vi "Read Frequency Response Analysis Data.vi"(8 "error in (no error)":errorcluster, 10 "Maximum Time (10000)":u32=10000, 11 "VISA resource name":refnum<visa-resource-name>) -> (0 "error out":errorcluster, 2 "Frequency Analysis Data":dbl[][](array[numeric]), 3 "VISA resource name out":refnum<visa-resource-name>)   [LabVIEW 2017, in "Agilent 2000 3000 X-Series.lvlib"]
doc: "Returns the frequency response analyze data.\nThe data is returned in four comma-separated columns of data for each step in the sweep: Frequency (Hz), Amplitude (Vpp), Gain (dB), and Phase (degree).\n\n<b>Note: </b>\nThis VI is applicable for 1000, 3000T, 3000G, 4000, 6000 X-Series."
uses:
  Agilent 2000 3000 X-Series.lvlib
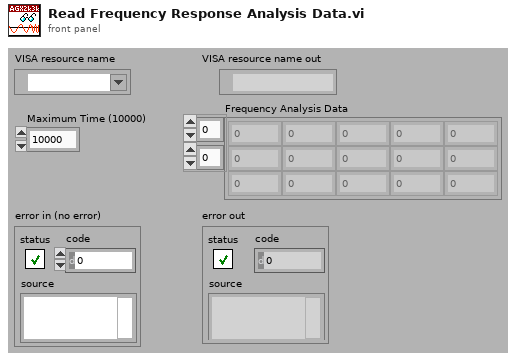
[diagram p1: front panel]
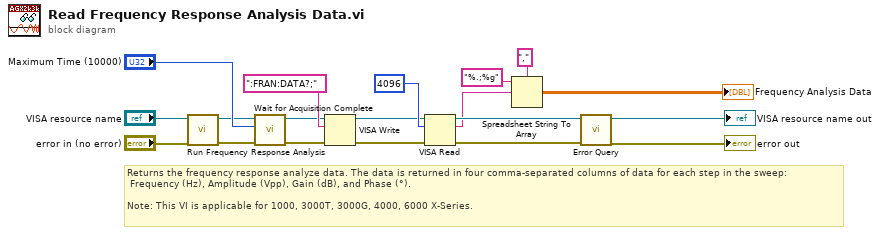
[diagram p0: block diagram]
diagram:
  # "Returns the frequency response analyze data. The data is returned in four comma-separated columns of data for each step in the sweep:\n Frequency (Hz), Amplitude (Vpp), Gain (dB), and Phase (°).\n\nNote: This VI is applicable for 1000, 3000T, 3000G, 4000, 6000 X-Series."
  n1 = call "Run Frequency Response Analysis.vi"("error in (no error)"="error in (no error)", "VISA resource name"="VISA resource name") -> ("error out"=w2:errorcluster, "VISA resource name out"=w1:refnum<visa-resource-name>)  [unwired: 8 in]
  n2 = call "Wait for Acquisition Complete.vi"("error in (no error)"=w2, "Maximum Time (10000)"="Maximum Time (10000)", "VISA resource name"=w1) -> ("error out"=w6:errorcluster, "VISA resource name out"=w7:refnum<visa-resource-name>)  [unwired: 7 in]
  n3 = VISA Write(VISA resource name=w7, write buffer=":FRAN:DATA?;", error in (no error)=w6) -> (VISA resource name out=w17:refnum<visa-resource-name>, error out=w16:errorcluster)  [unwired: 1 out]
  n4 = VISA Read(VISA resource name=w17, byte count=u32 4096, error in (no error)=w16) -> (VISA resource name out=w15:refnum<visa-resource-name>, read buffer=w11:string, error out=w14:errorcluster)  [unwired: 1 out]
  n5 = Spreadsheet String To Array(delimiter (Tab)=",", format string="%.;%g", spreadsheet string=w11) -> (array=→"Frequency Analysis Data":dbl[][])  [unwired: 1 in]
  n6 = call "Error Query.vi"("error in (no error)"=w14, "VISA resource name"=w15) -> ("error out"=→"error out":errorcluster, "VISA resource name out"=→"VISA resource name out":refnum<visa-resource-name>)  [unwired: 6 in, 2 out]
